vi "Length_12.vi"() -> ()   [LabVIEW 2020]
uses:
  Support/Controls/Clst_Initialize Input.ctl
  Support/Controls/Cmd_Var Data IO.ctl
  Support/Controls/Cmd_Mouse Popup.ctl
  Variables/Global_Cal Info.vi
panel:
  in  "Measured_ADJ2":string[][](table) caption="역(-)방향 지시값 (조정후)"
  in  "Measured_ADJ":string[][](table) caption="정(+)방향 지시값 (조정후)"
  in  "Measured 3":string[][](table) caption="되돌림오차측정"
  out "최소범위":string
  out "STD set":string[][](table) caption="○ 기준기 조합 (값)"
  in  "Measured 2":string[][](table) caption="역(-)방향 지시값"
  in  "표시방식":string(combo)
  out "단위":string
  out "최대범위":string
  in  "Spec 변경":bool
  in  "Random":bool
  out "Resolution":string[][](table) caption="Spec"
  out "Spec":string[][](table)
  out "제목":string
  out "에러 출력":errorcluster
  out "Condition":string[][](table) caption="2. 직선성 시험"
  in  "최소눈금":string(combo)
  in  "Measured":string[][](table) caption="정(+)방향 지시값"
  out "Load?":bool
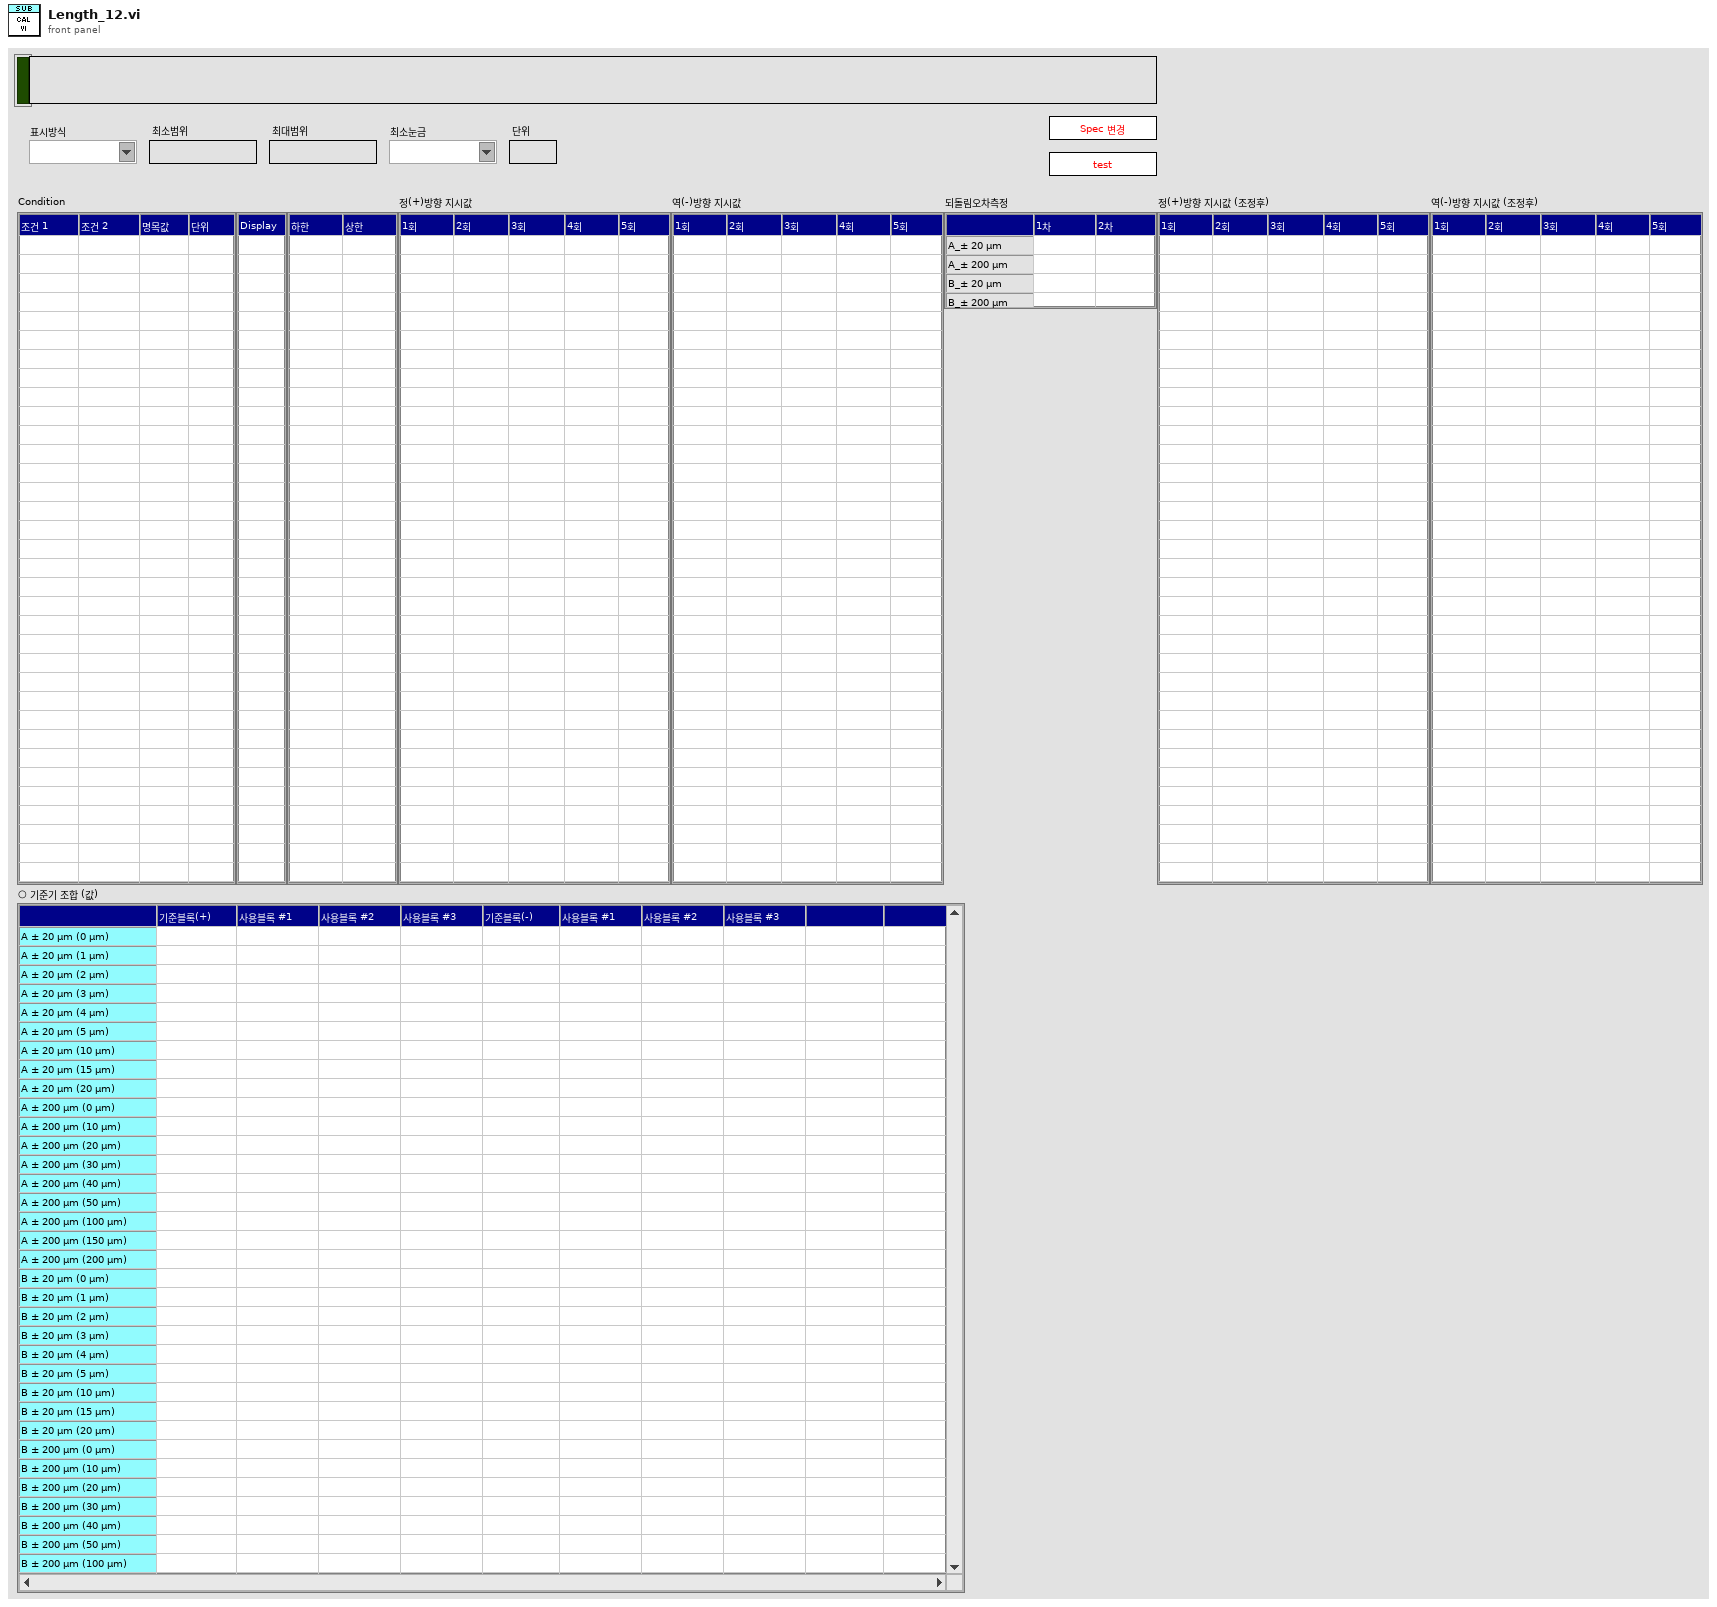
[diagram p1: front panel]
types:
  T1 = typedef "Cmd_Mouse Popup.ctl" = enum16{"활성화", "메뉴선택"}
  T2 = cluster{"Shift":bool, "Ctrl":bool, "Alt":bool, "Cmd":bool, "Opt":bool}
  T3 = typedef "Clst_Initialize Input.ctl" = cluster{"Initialize 1":cluster{"Condition":refnum<vi>[], "Spec":refnum<vi>[], "Measured":refnum<vi>[], "Resolution":refnum<vi>[], "Func_ext":string, "제목":refnum<vi>, "Measured_ADJ":refnum<vi>[]}, "Initialize 2":cluster{"문자열":refnum<vi>[], "콤보박스":refnum<vi>[], "링":refnum<vi>[], "열거형":refnum<vi>[], "테이블":refnum<vi>[], "여러열":refnum<vi>[], "디지털(DBL)":refnum<vi>[], "3D string":refnum<vi>[], "ctrl":refnum<vi>[], "boolean":refnum<vi>[]}}
  T4 = typedef "Cmd_Var Data IO.ctl" = enum16{"Condition", "Condition Default", "Condition_Temp", "Resolution", "Resolution Default", "Resolution Old", "Spec", "Spec Default", "Spec Old", "Spec Temp", "Result", "Result2", "Result3", "Result_Temp", "Result_ADJ", "Result_ADJ2", "STD1", "STD2", "STD3", "STD4", "STD5", "STD Temp", "CMC", "CMC Default"}
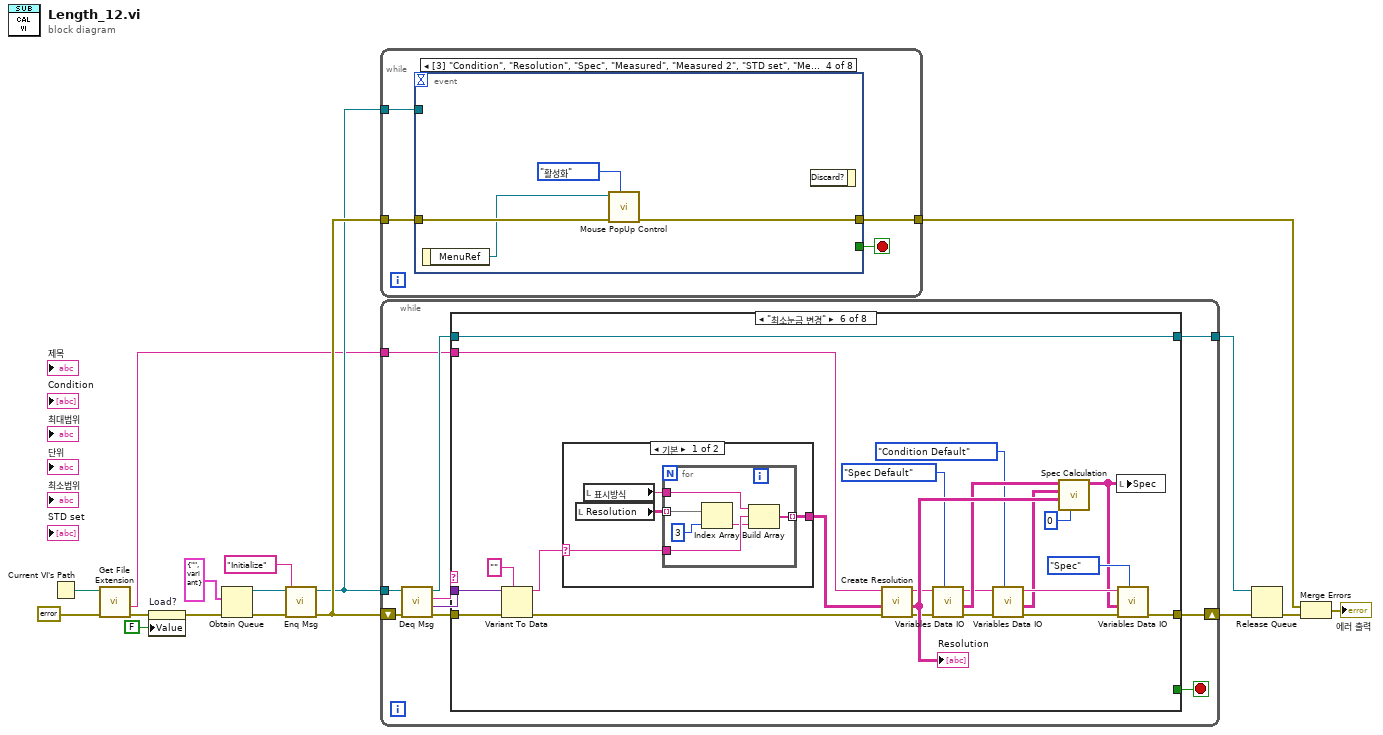
[diagram p0: block diagram]
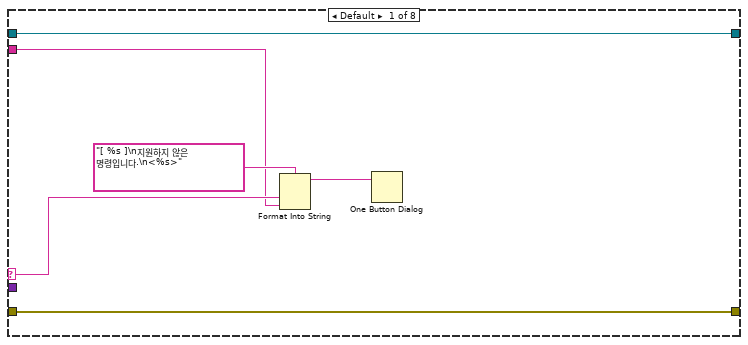
[diagram p2: hidden frame]
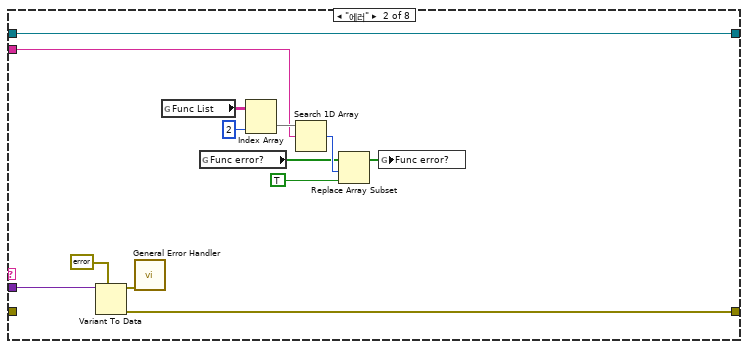
[diagram p3: hidden frame]
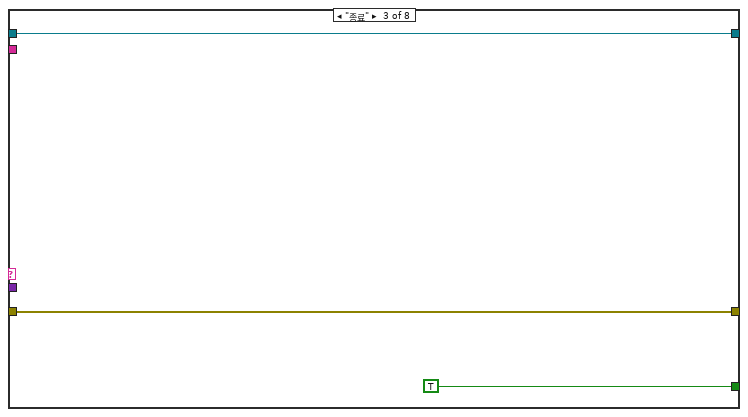
[diagram p4: hidden frame]
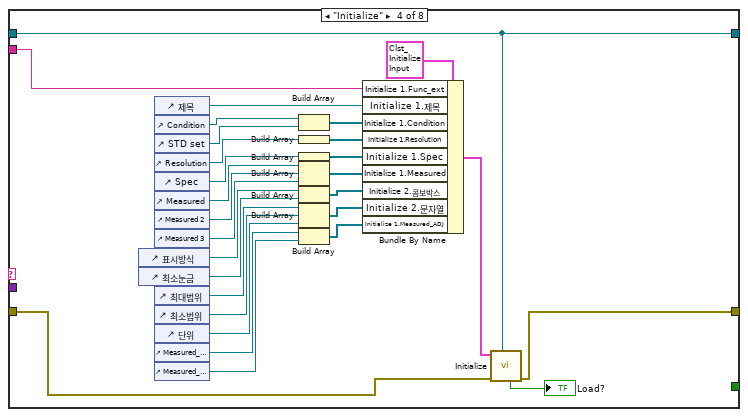
[diagram p5: hidden frame]
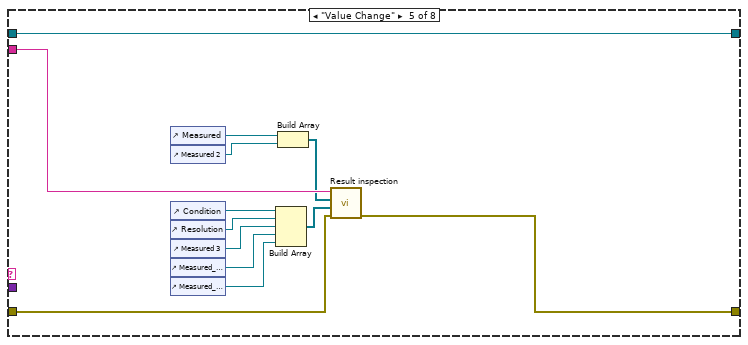
[diagram p6: hidden frame]
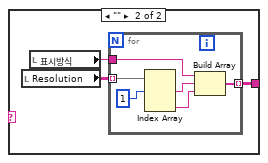
[diagram p7: hidden frame]
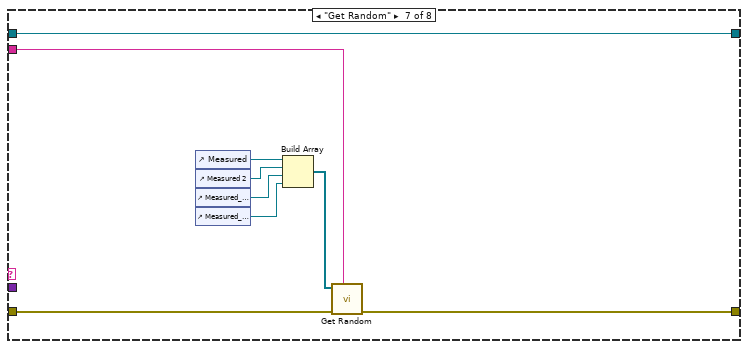
[diagram p8: hidden frame]
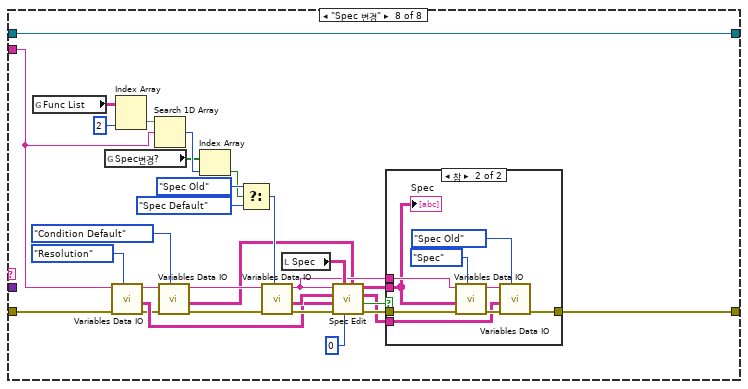
[diagram p9: hidden frame]
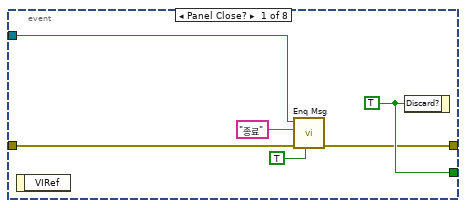
[diagram p11: hidden frame]
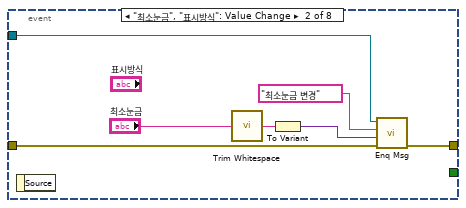
[diagram p12: hidden frame]
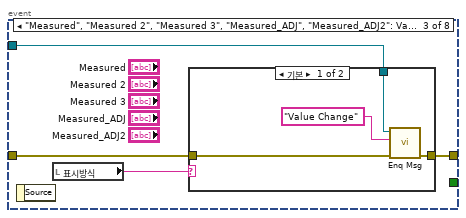
[diagram p13: hidden frame]
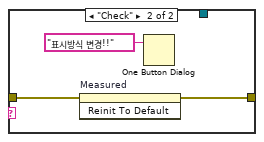
[diagram p14: hidden frame]
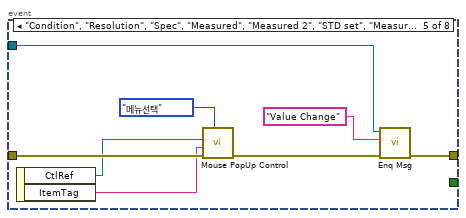
[diagram p15: hidden frame]
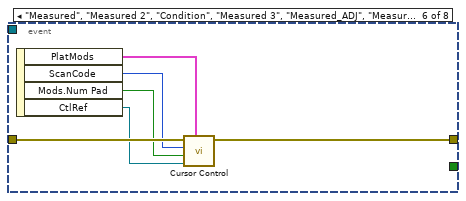
[diagram p16: hidden frame]
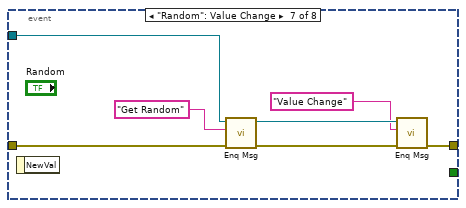
[diagram p17: hidden frame]
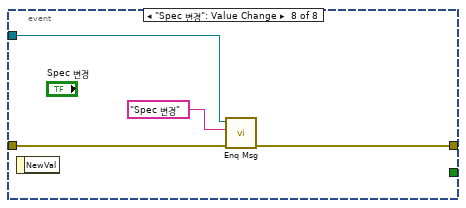
[diagram p18: hidden frame]
diagram:
  n1 = Current VI's Path() -> (path=w5:path)
  n2 = call <vilib>:"Get File Extension.vi"("error in (no error)"=errorcluster {"status"=FALSE, "code"=0, "source"=""} ("에러 상수"), "file"=w5) -> ("error out"=w3:errorcluster, "filename without extension"=w4:string)  [unwired: 5 in, 3 out]
  n3 = property on="Load?" class="Bool (엄격한)"(error in=w3, "Value"=FALSE ("Load?")) -> (error out=w2:errorcluster)  [unwired: 1 in, 1 out]
  n4 = Obtain Queue(element data type=cluster{"메세지":string, "값":variant} {"메세지"="", "값"=variant} ("Message Cluster"), error in (no error)=w2) -> (queue out=w14:refnum<queue>, error out=w16:errorcluster)  [unwired: 3 in, 1 out]
  n5 = call "Enq Msg.vi"("에러 입력(에러 없음)"=w16, "메세지"="Initialize", "큐 입력"=w14) -> ("에러 출력"=w15:errorcluster, "큐 출력"=w12:refnum<queue>)  [unwired: 7 in]
  n6 = while {
    tunnel: w15 -> [w19]
    tunnel: w12 -> [w20]
    tunnel: [w18] -> w9
    stop <- w21 stop-if-true
    n7 = event shown="[3] \"Condition\", \"Resolution\", \"Spec\", \"Measured\", \"Measured 2\", \"STD set\", \"Measured 3\", \"Measured_ADJ\", \"Measured_ADJ2\": 바로 가기 메뉴 활성화?" {
      selector: _ -> [_ _ _ _ _ _ _ _]
      dyn-events: _ -> [_ _ _ _ _ _ _ _]
      timeout: _ -> [_ _ _ _ _ _ _ _]
      tunnel: [w27 _ _ _ _ _ _ _] -> w21
      tunnel: w20 -> [w25 w33 w38 _ w50 _ w68 w72]
      tunnel: w19 -> [w26 w34 w36 w49 w57 w63 w69 w73]
      tunnel: [w23 w32 w37 w48 w51 w62 w64 w71] -> w18
      event Panel Close? {
        w27 = TRUE ("버림?")
        n8 = event-data() -> ()  [unwired: 1 in, 1 out]
        n9 = call "Enq Msg.vi"("우선순위 메시지?"=TRUE, "에러 입력(에러 없음)"=w26, "메세지"="종료", "큐 입력"=w25) -> ("에러 출력"=w23:errorcluster)  [unwired: 6 in, 1 out]
        n10 = event-data("Discard?"=w27) -> ()  [unwired: 1 in, 1 out]
      }
      event "최소눈금", "표시방식": Value Change {
        n11 = event-data() -> ()  [unwired: 1 in, 1 out]
        n12 = call <vilib>:"Trim Whitespace.vi"("string"="최소눈금") -> ("trimmed string"=w30:string)  [unwired: 1 in]
        n13 = To Variant(anything=w30) -> (Variant=w28:variant)
        n14 = call "Enq Msg.vi"("에러 입력(에러 없음)"=w34, "값"=w28, "메세지"="최소눈금 변경", "큐 입력"=w33) -> ("에러 출력"=w32:errorcluster)  [unwired: 6 in, 1 out]
      }
      event "Measured", "Measured 2", "Measured 3", "Measured_ADJ", "Measured_ADJ2": Value Change {
        n15 = event-data() -> ()  [unwired: 1 in, 1 out]
        n16 = local read "표시방식"() -> (w35:string)
        n17 = case shown="기본" w35 {
          tunnel: w38 -> [w42 _]
          tunnel: [w41 w43] -> w37
          tunnel: w36 -> [w40 w44]
          frame Default {
            n18 = call "Enq Msg.vi"("에러 입력(에러 없음)"=w40, "메세지"="Value Change", "큐 입력"=w42) -> ("에러 출력"=w41:errorcluster)  [unwired: 7 in, 1 out]
          }
          frame "Check" {
            n19 = invoke on="Measured" class="Tbl (엄격한)" method="Reinit To Default"(error in=w44) -> (error out=w43:errorcluster)  [unwired: 2 in, 2 out]
            n20 = One Button Dialog(message="표시방식 변경!!" ("메시지")) -> ()  [unwired: 1 in, 1 out]
          }
        }
      }
      event "Condition", "Resolution", "Spec", "Measured", "Measured 2", "STD set", "Measured 3", "Measured_ADJ", "Measured_ADJ2": Shortcut Menu Activation? {
        n21 = event-data() -> ("MenuRef"=w47:refnum<k9>)  [unwired: 1 in]
        n22 = call "Mouse PopUp Control.vi"("type"=Cmd_Mouse_Popup."활성화", "error in"=w49, "메뉴 참조"=w47) -> ("error out"=w48:errorcluster)  [unwired: 8 in]
        n23 = event-data() -> ()  [unwired: 2 in, 1 out]
      }
      event "Condition", "Resolution", "Spec", "Measured", "Measured 2", "STD set", "Measured 3", "Measured_ADJ", "Measured_ADJ2": Shortcut Menu Selection (User) {
        n24 = event-data() -> ("CtlRef"=w55:refnum<vi>, "ItemTag"=w54:string)  [unwired: 1 in]
        n25 = call "Mouse PopUp Control.vi"("type"=Cmd_Mouse_Popup."메뉴선택", "error in"=w57, "아이템 태그"=w54, "Tbl 참조 번호"=w55) -> ("error out"=w52:errorcluster)  [unwired: 7 in]
        n26 = call "Enq Msg.vi"("에러 입력(에러 없음)"=w52, "메세지"="Value Change", "큐 입력"=w50) -> ("에러 출력"=w51:errorcluster)  [unwired: 7 in, 1 out]
      }
      event "Measured", "Measured 2", "Condition", "Measured 3", "Measured_ADJ", "Measured_ADJ2": Key Down; "Measured", "Measured 2", "Condition", "Measured 3", "Measured_ADJ", "Measured_ADJ2": Key Repeat {
        n27 = event-data() -> ("PlatMods"=w58:T2, "ScanCode"=w61:i16, "Mods.Num Pad"=w60:bool, "CtlRef"=w59:refnum<vi>)  [unwired: 1 in]
        n28 = call "Cursor Control.vi"("플랫폼 조합키"=w58, "참조"=w59, "Num Pad"=w60, "ScanCode"=w61, "error in"=w63) -> ("error out"=w62:errorcluster)  [unwired: 5 in, 1 out]
      }
      event "Random": Value Change {
        n29 = event-data() -> ()  [unwired: 1 in, 1 out]
        n30 = call "Enq Msg.vi"("에러 입력(에러 없음)"=w69, "메세지"="Get Random", "큐 입력"=w68) -> ("에러 출력"=w67:errorcluster, "큐 출력"=w66:refnum<queue>)  [unwired: 7 in]
        n31 = call "Enq Msg.vi"("에러 입력(에러 없음)"=w67, "메세지"="Value Change", "큐 입력"=w66) -> ("에러 출력"=w64:errorcluster)  [unwired: 7 in, 1 out]
      }
      event "Spec 변경": Value Change {
        n32 = event-data() -> ()  [unwired: 1 in, 1 out]
        n33 = call "Enq Msg.vi"("에러 입력(에러 없음)"=w73, "메세지"="Spec 변경", "큐 입력"=w72) -> ("에러 출력"=w71:errorcluster)  [unwired: 7 in, 1 out]
      }
    }
  }
  n34 = while {
    shift-right: [w84] -> w11
    shift-left: w15 -> [w83]
    tunnel: w12 -> [w81]
    tunnel: [w76] -> w10
    tunnel: w4 -> [w75]
    stop <- w77 stop-if-true
    n35 = call "Deq Msg.vi"("에러 입력(에러 없음)"=w83, "큐 입력"=w81) -> ("에러 출력"=w82:errorcluster, "값"=w78:variant, "메세지"=w80:string, "큐 출력"=w79:refnum<queue>)  [unwired: 6 in]
    n36 = case shown="\"최소눈금 변경\"" w80 {
      selector: w80 -> [w86 _ _ _ _ _ _ _]
      tunnel: w82 -> [w90 _ w106 w115 w145 w170 w195 w222]
      tunnel: [w90 w100 w106 w113 w147 w163 w196 w225] -> w84
      tunnel: w79 -> [w89 w99 w104 w121 w148 w171 w199 w229]
      tunnel: w78 -> [_ w101 _ _ _ w169 _ _]
      tunnel: [_ _ TRUE ("버림?") _ _ _ _ _] -> w77
      tunnel: [w89 w99 w104 w121 w148 w171 w199 w229] -> w76
      tunnel: w75 -> [w85 w91 _ w122 w146 w167 w194 w207]
      frame Default {
        n37 = Format Into String(format string="[ %s ]\n지원하지 않은 명령입니다.\n<%s>" ("메시지"), w86, w85) -> (resulting string=w87:string)  [unwired: 2 in, 1 out]
        n38 = One Button Dialog(message=w87) -> ()  [unwired: 1 in, 1 out]
      }
      frame "에러" {
        n39 = Variant To Data(type=errorcluster {"status"=FALSE, "code"=0, "source"=""} ("에러 출력"), Variant=w101) -> (data=w103:errorcluster, error out=w100:errorcluster)  [unwired: 1 in]
        n40 = call <vilib>:"General Error Handler.vi"("error in (no error)"=w103) -> ()  [unwired: 10 in, 5 out]
        n41 = global read "Global_Cal Info.vi" "Func List"() -> (w93:string[][])
        n42 = global read "Global_Cal Info.vi" "Func error?"() -> (w96:bool[])
        n43 = Index Array(array=w93, index (col)=2 ("비활성화된 인덱스 (열)")) -> (element=w94:string[])  [unwired: 1 in]
        n44 = Search 1D Array(1D array=w94, element=w91) -> (index of element=w97:i32)  [unwired: 1 in]
        n45 = Replace Array Subset(array=w96, new element=TRUE ("새 원소/부분배열"), index=w97) -> (w98:bool[])
        n46 = global write "Global_Cal Info.vi" "Func error?"(w98) -> ()
      }
      frame "종료" {
      }
      frame "Initialize" {
        n47 = control-ref of="표시방식"() -> (w120:refnum<vi>)
        n48 = control-ref of="최소눈금"() -> (w129:refnum<vi>)
        n49 = control-ref of="제목"() -> (w127:refnum<vi>)
        n50 = control-ref of="Condition"() -> (w133:refnum<vi>)
        n51 = control-ref of="STD set"() -> (w111:refnum<vi>)
        n52 = control-ref of="Resolution"() -> (w123:refnum<vi>)
        n53 = control-ref of="Spec"() -> (w126:refnum<vi>)
        n54 = control-ref of="Measured"() -> (w130:refnum<vi>)
        n55 = control-ref of="Measured 2"() -> (w116:refnum<vi>)
        n56 = control-ref of="Measured 3"() -> (w112:refnum<vi>)
        n57 = control-ref of="최대범위"() -> (w114:refnum<vi>)
        n58 = control-ref of="최소범위"() -> (w117:refnum<vi>)
        n59 = control-ref of="단위"() -> (w119:refnum<vi>)
        n60 = control-ref of="Measured_ADJ"() -> (w110:refnum<vi>)
        n61 = control-ref of="Measured_ADJ2"() -> (w109:refnum<vi>)
        n62 = Build Array(w133, w111) -> (w132:refnum<vi>[])
        n63 = Build Array(w123) -> (w124:refnum<vi>[])
        n64 = Build Array(w126) -> (w125:refnum<vi>[])
        n65 = Build Array(w130, w116, w112) -> (w131:refnum<vi>[])
        n66 = Build Array(w120, w129) -> (w128:refnum<vi>[])
        n67 = Build Array(w114, w117, w119) -> (w118:refnum<vi>[])
        n68 = Build Array(w110, w109) -> (w108:refnum<vi>[])
        n69 = Bundle By Name(cluster=T3 {"Initialize 1"={"Condition"=[], "Spec"=[], "Measured"=[], "Resolution"=[], "Func_ext"="", "제목"=refnum, "Measured_ADJ"=[]}, "Initialize 2"={"문자열"=[], "콤보박스"=[], "링"=[], "열거형"=[], "테이블"=[], "여러열"=[], "디지털(DBL)"=[], "3D string"=[], "ctrl"=[], "boolean"=[]}} ("입력 클러스터"), "Initialize 1.Func_ext"=w122, "Initialize 1.제목"=w127, "Initialize 1.Condition"=w132, "Initialize 1.Resolution"=w124, "Initialize 1.Spec"=w125, "Initialize 1.Measured"=w131, "Initialize 2.콤보박스"=w128, "Initialize 2.문자열"=w118, "Initialize 1.Measured_ADJ"=w108) -> (w134:T3)
        n70 = call "Initialize.vi"("큐 입력"=w121, "error in"=w115, "입력 클러스터"=w134) -> ("error out"=w113:errorcluster, "Load?"=→"Load?":bool)  [unwired: 5 in, 2 out]
      }
      frame "Value Change" {
        n71 = control-ref of="Measured"() -> (w144:refnum<vi>)
        n72 = control-ref of="Measured 2"() -> (w142:refnum<vi>)
        n73 = control-ref of="Condition"() -> (w140:refnum<vi>)
        n74 = control-ref of="Resolution"() -> (w138:refnum<vi>)
        n75 = control-ref of="Measured 3"() -> (w139:refnum<vi>)
        n76 = control-ref of="Measured_ADJ"() -> (w137:refnum<vi>)
        n77 = control-ref of="Measured_ADJ2"() -> (w136:refnum<vi>)
        n78 = Build Array(w140, w138, w139, w137, w136) -> (w141:refnum<vi>[])
        n79 = Build Array(w144, w142) -> (w143:refnum<vi>[])
        n80 = call "Result inspection.vi"("error in"=w145, "Ref. Data (excluded)"=w141, "Ref. Data (Inspection)"=w143, "Func ext"=w146) -> ("error out"=w147:errorcluster)  [unwired: 4 in, 3 out]
      }
      frame "최소눈금 변경" {
        n81 = Variant To Data(error in=w170, type="", Variant=w169) -> (data=w156:string, error out=w158:errorcluster)
        n82 = case shown="기본" w156 {
          selector: w156 -> [w172 _]
          tunnel: [w175 w184] -> w157
          frame Default {
            n83 = local read "Resolution"() -> (w174:string[][])
            n84 = local read "표시방식"() -> (w173:string)
            n85 = for {
              tunnel: w174 -> [w181] mode=indexing
              tunnel: w172 -> [w180]
              tunnel: [w178] -> w175 mode=indexing
              tunnel: w173 -> [w177]
              n86 = Index Array(array=w181, index=3 ("인덱스")) -> (element=w179:string)
              n87 = Build Array(w177, w180, w179) -> (w178:string[])
            }
          }
          frame "" {
            n88 = local read "Resolution"() -> (w183:string[][])
            n89 = local read "표시방식"() -> (w182:string)
            n90 = for {
              tunnel: w183 -> [w190] mode=indexing
              tunnel: [w189] -> w184 mode=indexing
              tunnel: w182 -> [w188]
              n91 = Index Array(array=w190, index #1=1 ("인덱스")) -> (element #1=w186:string, element #3=w185:string)  [unwired: 2 in, 1 out]
              n92 = Build Array(w188, w186, w185) -> (w189:string[])
            }
          }
        }
        n93 = call "Create Resolution.vi"("에러 입력(에러 없음)"=w158, "Resolution"=w157, "Func_ext"=w167) -> ("에러 출력"=w161:errorcluster, "Resolution Out"=w164:string[][], "Func_ext 출력"=w160:string)  [unwired: 6 in]
        "Resolution" <- w164
        n94 = call "Variables Data IO.vi"("Select"=Cmd_Var_Data_IO."Spec Default", "error in"=w161, "Func_ext"=w160) -> ("error out"=w153:errorcluster, "Data Out"=w159:string[][], "Func_ext Out"=w155:string)  [unwired: 6 in]
        n95 = call "Variables Data IO.vi"("Select"=Cmd_Var_Data_IO."Condition Default", "error in"=w153, "Func_ext"=w155) -> ("error out"=w152:errorcluster, "Data Out"=w150:string[][], "Func_ext Out"=w154:string)  [unwired: 6 in]
        n96 = call "Spec Calculation.vi"("기준값 열번호"=0 ("열번호(기준값)"), "Resolution"=w164, "Condition in"=w150, "Spec Default"=w159) -> ("Spec out"=w149:string[][])  [unwired: 6 in, 1 out]
        n97 = local write "Spec"(w149) -> ()
        n98 = call "Variables Data IO.vi"("Select"=Cmd_Var_Data_IO."Spec", "error in"=w152, "Data In"=w149, "Func_ext"=w154) -> ("error out"=w163:errorcluster)  [unwired: 5 in, 2 out]
      }
      frame "Get Random" {
        n99 = control-ref of="Measured"() -> (w198:refnum<vi>)
        n100 = control-ref of="Measured 2"() -> (w193:refnum<vi>)
        n101 = control-ref of="Measured_ADJ"() -> (w192:refnum<vi>)
        n102 = control-ref of="Measured_ADJ2"() -> (w191:refnum<vi>)
        n103 = Build Array(w198, w193, w192, w191) -> (w197:refnum<vi>[])
        n104 = call "Get Random.vi"("Func_Ext"=w194, "에러 입력"=w195, "Meas"=w197) -> ("에러 출력"=w196:errorcluster)  [unwired: 7 in, 1 out]
      }
      frame "Spec 변경" {
        n105 = global read "Global_Cal Info.vi" "Func List"() -> (w212:string[][])
        n106 = global read "Global_Cal Info.vi" "Spec변경?"() -> (w208:bool[])
        n107 = call "Variables Data IO.vi"("Select"=Cmd_Var_Data_IO."Resolution", "error in"=w222, "Func_ext"=w207) -> ("error out"=w205:errorcluster, "Data Out"=w216:string[][], "Func_ext Out"=w203:string)  [unwired: 6 in]
        n108 = Index Array(array=w212, index (col)=2 ("비활성화된 인덱스 (열)")) -> (element=w210:string[])  [unwired: 1 in]
        n109 = Search 1D Array(1D array=w210, element=w207) -> (index of element=w209:i32)  [unwired: 1 in]
        n110 = call "Variables Data IO.vi"("Select"=Cmd_Var_Data_IO."Condition Default", "error in"=w205, "Func_ext"=w203) -> ("error out"=w204:errorcluster, "Data Out"=w200:string[][], "Func_ext Out"=w202:string)  [unwired: 6 in]
        n111 = Index Array(array=w208, index=w209) -> (element=w213:bool)
        n112 = Select(t=Cmd_Var_Data_IO."Spec Old" ("Select"), s=w213, f=Cmd_Var_Data_IO."Spec Default" ("Select")) -> (s? t:f=w206:T4)
        n113 = call "Variables Data IO.vi"("Select"=w206, "error in"=w204, "Func_ext"=w202) -> ("error out"=w224:errorcluster, "Data Out"=w217:string[][], "Func_ext Out"=w218:string)  [unwired: 6 in]
        n114 = local read "Spec"() -> (w219:string[][])
        n115 = call "Spec Edit.vi"("Condition"=w200, "열번호(기준값)"=0, "Spec Value"=w219, "에러 입력(에러 없음)"=w224, "Resolution"=w216, "Spec Default"=w217, "Func_ext"=w218) -> ("에러 출력"=w226:errorcluster, "변경?"=w227:bool, "Spec Default out"=w221:string[][], "Spec 출력"=w228:string[][])  [unwired: 1 in]
        n116 = case shown="참" w227 {
          tunnel: w228 -> [_ w236]
          tunnel: w226 -> [w230 w239]
          tunnel: [w230 w234] -> w225
          tunnel: w218 -> [_ w237]
          tunnel: w221 -> [_ w232]
          frame False {
          }
          frame True {
            n117 = call "Variables Data IO.vi"("Select"=Cmd_Var_Data_IO."Spec", "error in"=w239, "Data In"=w236, "Func_ext"=w237) -> ("error out"=w235:errorcluster, "Func_ext Out"=w233:string)  [unwired: 5 in, 1 out]
            n118 = call "Variables Data IO.vi"("Select"=Cmd_Var_Data_IO."Spec Old", "error in"=w235, "Data In"=w232, "Func_ext"=w233) -> ("error out"=w234:errorcluster)  [unwired: 5 in, 2 out]
            "Spec" <- w236
          }
        }
      }
    }
  }
  n119 = Release Queue(queue=w10, error in (no error)=w11) -> (error out=w8:errorcluster)  [unwired: 1 in, 2 out]
  n120 = Merge Errors(w9, w8) -> (→"에러 출력":errorcluster)
